vi "PH_Beckhoff.Ping Hardware.vi"(0 "i ref in":refnum<vi>, 5 "error in":errorcluster) -> (14 "i ref out":refnum<vi>, 19 "error out":errorcluster)   [LabVIEW 2014, in "PH_Beckhoff.lvlib"]
doc: "This VI tries to ping the hardware and sets the results to own attributes and related GUI elements."
uses:
  PH_Beckhoff.lvlib
  CSCore/BaseProcess/BaseProcess.lvlib
  non_GPL/instr.lib/Beckhoff/Beckhoff - Driver np.lvlib
  PH_Common/PH_Common.lvlib
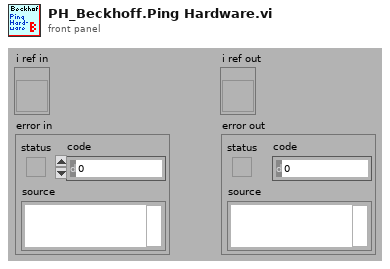
[diagram p1: front panel]
types:
  T1 = typedef "PH_Beckhoff.lvlib/PH_Beckhoff.i attribute.ctl" = cluster{"GUI Refs":T2, "operation?":bool, "Default Prdc Interval":i32, "Connection":T3, "AMS Net ID":T4, "Klemmencluster: # of":T5, "Values":T6, "IP":string, "Description":string, "configured?":bool, "Change Manager":cluster{"Detemination wanted?":bool, "Values changed at":cluster{"Sonderklemmen Inputs":i32[], "Analog Inputs":i32[], "Analog Outputs":i32[], "Digital Inputs":i32[], "Digital Outputs":i32[]}}, "Difference to handle an analog input as change":u32}
  T2 = typedef "PH_Beckhoff.lvlib/PH_Beckhoff.GUI Refs.ctl" = cluster{"ADS Error":refnum<vi>, "Values":refnum<vi>, "configured?":refnum<vi>, "Connection":refnum<vi>, "IP":refnum<vi>, "Prdc Int [ms]":refnum<vi>}
  T3 = typedef "PH_Beckhoff.lvlib/PH_Beckhoff.Connectivity.ctl" = cluster{"DLL?":bool, "Port?":bool, "Client?":bool, "Ping?":bool, "unsuccessful Pings":u32}
  T4 = typedef "Beckhoff - Driver np.lvlib/Beckhoff Access.ctl" = cluster{"DLL path":path, "AMS Net ID":cluster{"1st # of IP":u8, "2nd # of IP":u8, "3rd # of IP":u8, "4th # of IP":u8, "In Port":u8, "Out Port":u8}}
  T5 = typedef "Beckhoff - Driver np.lvlib/Klemmendeclarer.ctl" = cluster{"Offset due to Sonderklemms":u32, "analog Inputs":u32, "analog Outputs":u32, "digital Input Bits":u32, "digital Output Bits":u32}
  T6 = typedef "PH_Beckhoff.lvlib/PH_Beckhoff.Values.ctl" = cluster{"Sonderklemmen Inputs":T7, "Analog Inputs":T8, "Analog Outputs":T10, "Digital Inputs":T11, "Digital Outputs":T12}
  T7 = typedef "PH_Beckhoff.lvlib/PH_Beckhoff.Sonderklemmen Inputs.ctl" = cluster{"Total Length":u32, "Name":string, "Value":u64, "Quality":bool, "Service ID":i32, "Offset":u32, "Length":u32}[]
  T8 = typedef "PH_Beckhoff.lvlib/PH_Beckhoff.Analog Inputs.ctl" = cluster{"Name":string, "Value":u32, "Quality":bool, "Service ID":i32, "Sca Type":T9}[]
  T9 = typedef "PH_Beckhoff.lvlib/PH_Beckhoff.Scaling Type.ctl" = enum16{"none", "0 ... 15 Bit -> 0 ... 5", "0 ... 15 Bit -> 0 ... 10", "0 ... 15 Bit -> 0 ... 25", "0 ... 15 Bit -> 4 ... 20", "0 ... 15 Bit -> 0 ... 1", "0 ... 15 Bit -> 0 ... 20000", "0 ... 15 Bit -> 0 ... 24000"}
  T10 = typedef "PH_Beckhoff.lvlib/PH_Beckhoff.Analog Outputs.ctl" = cluster{"Name":string, "Value":u32, "Quality":bool, "Wanted Value":u32, "Service ID":i32, "Sca Type":T9}[]
  T11 = typedef "PH_Beckhoff.lvlib/PH_Beckhoff.Digital Inputs.ctl" = cluster{"Name":string, "Value":bool, "Quality":bool, "Service ID":i32, "inverted?":bool}[]
  T12 = typedef "PH_Beckhoff.lvlib/PH_Beckhoff.Digital Outputs.ctl" = cluster{"Name":string, "Value":bool, "Quality":bool, "Wanted Value":bool, "Service ID":i32, "inverted?":bool}[]
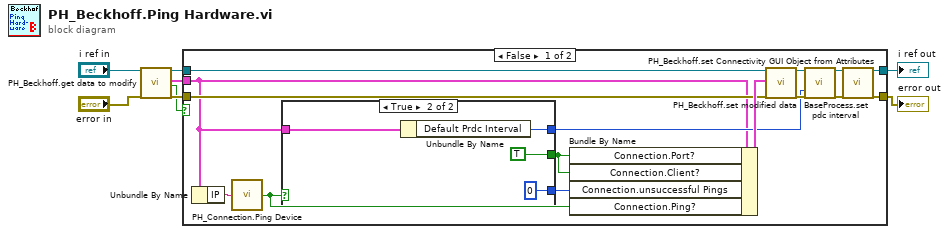
[diagram p0: block diagram]
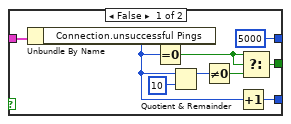
[diagram p2: hidden frame]
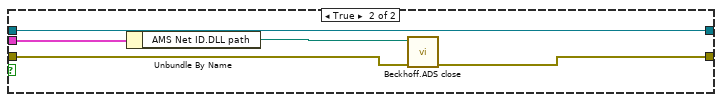
[diagram p3: hidden frame]
diagram:
  n1 = call "PH_Beckhoff.get data to modify.vi"("i ref in"="i ref in", "error in (no error)"="error in") -> ("i ref out"=w5:refnum<vi>, "i attribute"=w3:T1, "timed out"=w2:bool, "error out"=w4:errorcluster)  [unwired: 14 in]
  n2 = case shown="False" w2 {
    tunnel: w4 -> [w16 w40]
    tunnel: [w12 w39] -> w7
    tunnel: w5 -> [w23 w41]
    tunnel: [w14 w41] -> w6
    tunnel: w3 -> [w11 w38]
    frame False {
      n3 = Unbundle By Name(w11) -> ("IP"=w10:string)
      n4 = call "PH_Connection.Ping Device.vi"("IP"=w10) -> ("successfully pinged?"=w9:bool)
      n5 = case shown="True" w9 {
        tunnel: w11 -> [w32 w36]
        tunnel: [5000 ("Default Prdc Interval") w35] -> w18
        tunnel: [w31 u32 0] -> w20
        tunnel: [w26 TRUE] -> w17
        frame False {
          n6 = Unbundle By Name(w32) -> ("Connection.unsuccessful Pings"=w27:u32)
          n7 = Equal To 0?(x=w27) -> (x = 0?=w25:bool)
          n8 = Quotient & Remainder(x=w27, y=u32 10) -> (x-y*floor(x/y)=w28:u32)  [unwired: 1 out]
          n9 = Not Equal To 0?(x=w28) -> (x != 0?=w24:bool)
          n10 = Increment(x=w27) -> (x+1=w31:u32)
          n11 = Select(t=w25, s=w25, f=w24) -> (s? t:f=w26:bool)
        }
        frame True {
          n12 = Unbundle By Name(w36) -> ("Default Prdc Interval"=w35:i32)
        }
      }
      n13 = Bundle By Name(cluster=w11, "Connection.Port?"=w17, "Connection.Client?"=w17, "Connection.unsuccessful Pings"=w20, "Connection.Ping?"=w9) -> (w22:T1)
      n14 = call "PH_Beckhoff.set modified data.vi"("i ref in"=w23, "i attribute"=w22, "error in (no error)"=w16) -> ("i ref out"=w19:refnum<vi>, "error out"=w21:errorcluster)  [unwired: 15 in]
      n15 = call "BaseProcess.set pdc interval.vi"("i ref in"=w19, "PeriodicInterval [ms]"=w18, "error in (no error)"=w21) -> ("i ref out"=w15:refnum<vi>, "error out"=w13:errorcluster)  [unwired: 14 in, 1 out]
      n16 = call "PH_Beckhoff.set Connectivity GUI Object from Attributes.vi"("i ref in"=w15, "error in"=w13) -> ("i ref out"=w14:refnum<vi>, "error out"=w12:errorcluster)  [unwired: 16 in]
    }
    frame True {
      n17 = Unbundle By Name(w38) -> ("AMS Net ID.DLL path"=w37:path)
      n18 = call "Beckhoff.ADS close.vi"("error in"=w40, "path in"=w37) -> ("error out"=w39:errorcluster)  [unwired: 4 in, 1 out]
    }
  }
  "error out" <- w7
  "i ref out" <- w6
